vi "SEA_9811_Start.vi"(8 "error in (no error)":errorcluster, 11 "SEA9811_RT_data in":T1 {"Tx"."Tx Refs (Data,Trig)"."Data Reference" format="%.0x"}) -> (0 "error out":errorcluster, 3 "SEA9811_RT_data out":T1 {"Tx"."Tx Refs (Data,Trig)"."Data Reference" format="%.0x"})   [LabVIEW 2015]
uses:
  Typdefs/SEA9811_RT_data_cluster.ctl
  <userlib>/_FPGA Interface Advanced Tools/FPGA Interface Base/FPGA Interface Base.lvclass
  Typdefs/FPGA ref.ctl
  Typdefs/channel.ctl
  Typdefs/received word.ctl
  Typdefs/SEA9811_FPGA_FP_Addresses.ctl
  <vilib>/NI Veristand/Custom Device API/Block Data Reference.ctl
  <vilib>/NI Veristand/Custom Device API/Data Reference.ctl
  <userlib>/_FPGA Interface Advanced Tools/FPGA Interface Base/FPGA Write By Name - Boolean.vi
  <vilib>/NI VeriStand/Custom Device API/Custom Device API.lvlib
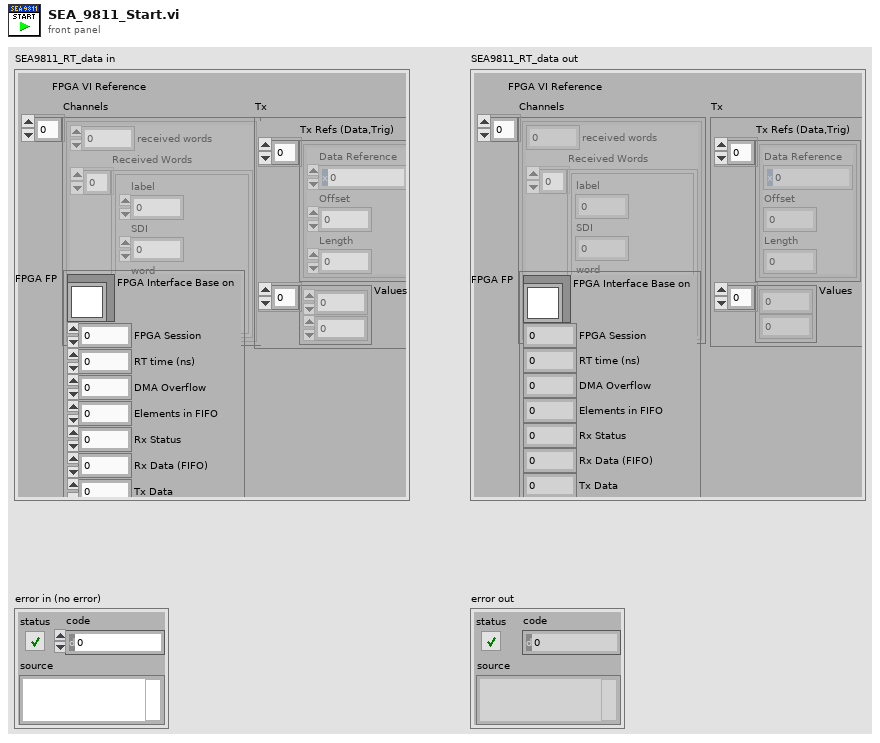
[diagram p1: front panel]
types:
  T1 = typedef "SEA9811_RT_data_cluster.ctl" = cluster{"FPGA VI Reference":T2, "Channels":T3[], "FPGA FP":T5, "Tx":cluster{"Tx Refs (Data,Trig)":T6[], "Values":dbl[]}}
  T2 = typedef "FPGA ref.ctl" = refnum<k20>
  T3 = typedef "channel.ctl" = cluster{"received words":u32, "Received Words":T4[]}
  T4 = typedef "received word.ctl" = cluster{"label":u8, "SDI":u8, "word":u32, "timestamp":dbl}
  T5 = typedef "SEA9811_FPGA_FP_Addresses.ctl" = cluster{"FPGA Interface Base on":refnum<class "FPGA Interface Base.lvclass">, "FPGA Session":u32, "RT time (ns)":u32, "DMA Overflow":u32, "Elements in FIFO":u32, "Rx Status":u32, "Rx Data (FIFO)":u32, "Tx Data":u32, "Transmit Data":u32}
  T6 = typedef "Custom Device API.lvlib/Block Data Reference.ctl" = cluster{"Data Reference":T7, "Offset":u64, "Length":u64}
  T7 = typedef "Custom Device API.lvlib/Data Reference.ctl" = i32
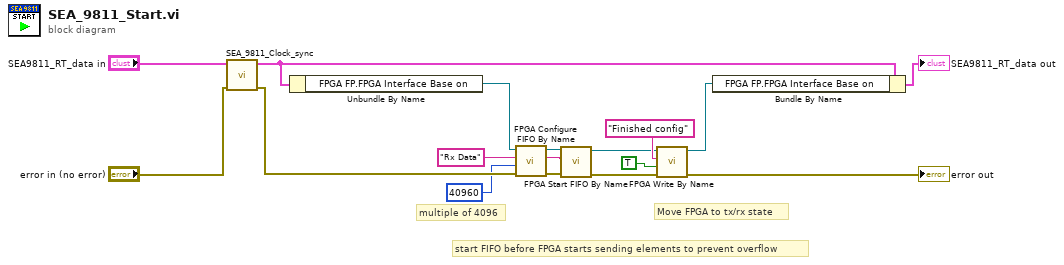
[diagram p0: block diagram]
diagram:
  w2 = "Rx Data" ("Control")
  # "start FIFO before FPGA starts sending elements to prevent overflow"
  # "multiple of 4096"
  # "Move FPGA to tx/rx state"
  n1 = call "SEA_9811_Clock_sync.vi"("error in (no error)"="error in (no error)", "SEA9811_RT_data in"="SEA9811_RT_data in") -> ("error out"=w6:errorcluster, "SEA9811_RT_data out"=w10:T1)  [unwired: 8 in]
  n2 = Unbundle By Name(w10) -> ("FPGA FP.FPGA Interface Base on"=w4:refnum<class "FPGA Interface Base.lvclass">)
  n3 = call <userlib>:"FPGA Configure FIFO By Name.vi"("error in (no error)"=w6, "Depth"=u64 40960, "FIFO"=w2, "FPGA Session In"=w4) -> ("error out"=w8:errorcluster, "FPGA Session Out"=w7:refnum<class "FPGA Interface Base.lvclass">)  [unwired: 6 in]
  n4 = call <userlib>:"FPGA Start FIFO By Name.vi"("error in (no error)"=w8, "FIFO"=w2, "FPGA Session In"=w7) -> ("error out"=w5:errorcluster, "FPGA Session Out"=w3:refnum<class "FPGA Interface Base.lvclass">)  [unwired: 7 in]
  n5 = call-poly <userlib>:"FPGA Write By Name.vi"("error in (no error)"=w5, "Value"=TRUE ("Finished config"), "Control"="Finished config", "FPGA Session In"=w3) -> ("error out"=→"error out":errorcluster, "FPGA Session Out"=w13:refnum<class "FPGA Interface Base.lvclass">)  [unwired: 6 in]
  n6 = Bundle By Name(cluster=w10, "FPGA FP.FPGA Interface Base on"=w13) -> (→"SEA9811_RT_data out":T1)
